vi "Configure Channel (Volt Log).vi"(0 "VISA resource name":refnum<visa-resource-name>, 1 "Scaling":T2={"Floating Point Position (2)"=2, "Lower Scaling (1.00E+0)"=1.0, "Upper Scaling (1.00E+2)"=100.0, "Unit Character (\"\")"=""} {"Upper Scaling (1.00E+2)" min=1e-15 max=1000000000000000.0 format="%.2e"; "Lower Scaling (1.00E+0)" min=1e-15 max=1000000000000000.0 format="%.2e"; "Floating Point Position (2)" min=1 max=2 step=1}, 5 "Channel (0001)":string="0001", 7 "Enable Channel (True)":bool=TRUE, 9 "Range And Span":T1={"Volt Range (4 : 2V)"=4, "Enable Span (False)"=FALSE, "Lower Span (2.0000)"=-2.0, "Upper Span (2.0000)"=2.0, "Bias (0)"=0.0} {"Upper Span (2.0000)" min=-99999.0 max=99999.0 step=1.0 format="%_5g"; "Lower Span (2.0000)" min=-99999.0 max=99999.0 step=1.0 format="%_5g"; "Volt Range (4 : 2V)" items=["20mV", "60mV", "200mV", "1V", "2V", "6V", "20V", "50V"]}, 11 "error in (no error)":errorcluster, 12 "Calculation (0: Log Input)":u16(ring) items=["Log Input", "Pseudo-log Input", "Linear-log Input"]) -> (4 "VISA resource name out":refnum<visa-resource-name>, 6 "Channel":string, 15 "error out":errorcluster)   [LabVIEW 2020, in "Yokogawa GX Series.lvlib"]
doc: "Sets the input range as voltage.\n\nCommand: SRangeAI"
uses:
  <instrlib>/Yokogawa GX Series/Yokogawa GX Series.lvlib
  <instrlib>/Yokogawa GX Series/Private/Volt Range.vi
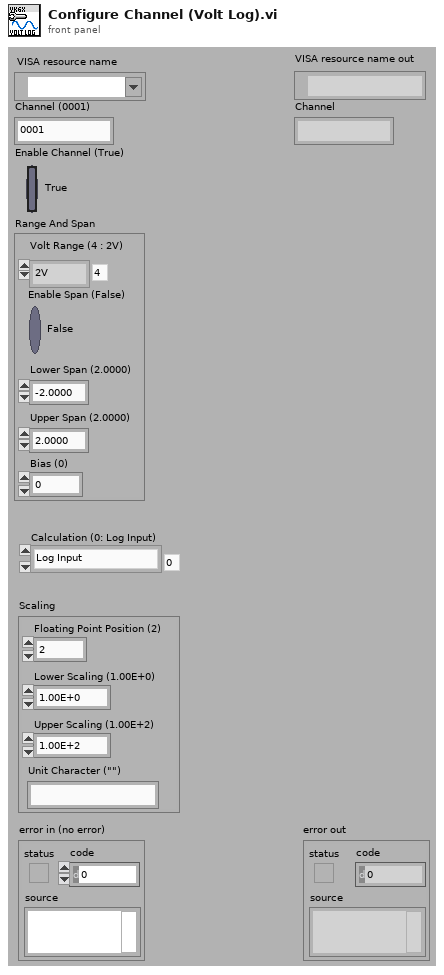
[diagram p1: front panel]
types:
  T1 = cluster{"Volt Range (4 : 2V)":i32, "Enable Span (False)":bool, "Lower Span (2.0000)":dbl, "Upper Span (2.0000)":dbl, "Bias (0)":dbl}
  T2 = cluster{"Floating Point Position (2)":i32, "Lower Scaling (1.00E+0)":dbl, "Upper Scaling (1.00E+2)":dbl, "Unit Character (\"\")":string}
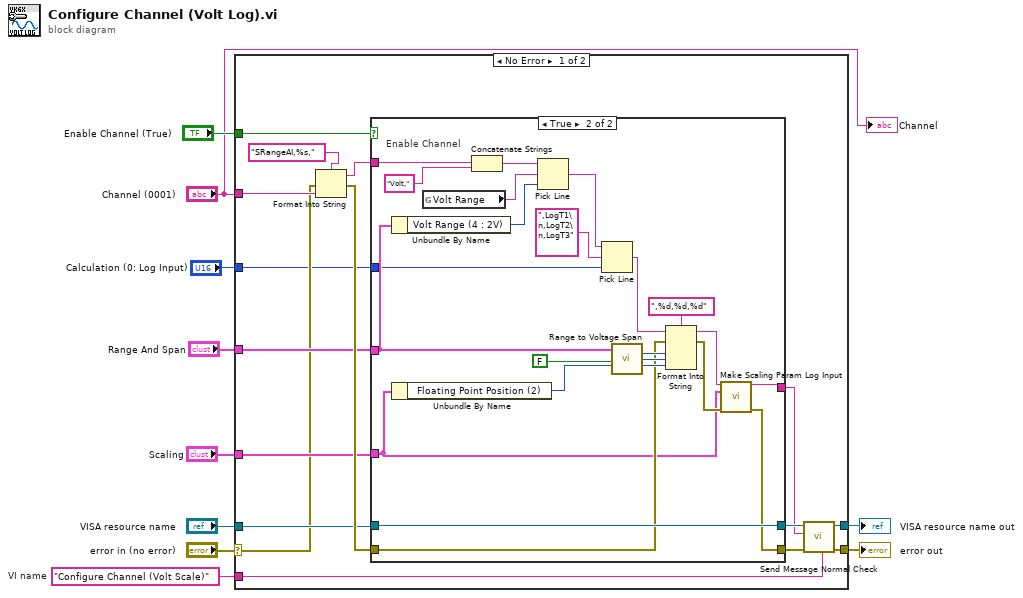
[diagram p0: block diagram]
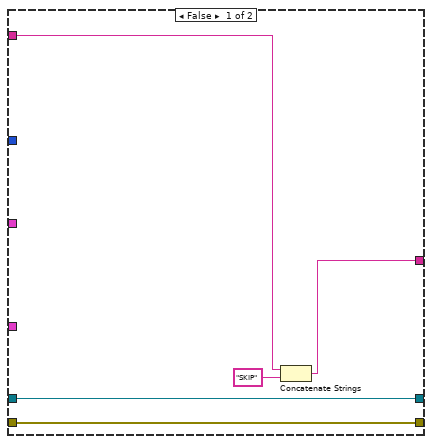
[diagram p2: hidden frame]
diagram:
  w6 = "Configure Channel (Volt Scale)"  # VI name
  n1 = case shown="No Error" "error in (no error)" {
    selector: "error in (no error)" -> [w12 w55]
    tunnel: "VISA resource name" -> [w23 w56]
    tunnel: "Scaling" -> [w22 _]
    tunnel: [w19 w56] -> w8
    tunnel: [w18 w55] -> w7
    tunnel: w6 -> [w16 _]
    tunnel: "Range And Span" -> [w15 _]
    tunnel: "Enable Channel (True)" -> [w14 _]
    tunnel: "Channel (0001)" -> [w13 _]
    tunnel: "Calculation (0: Log Input)" -> [w11 _]
    frame No Error {
      n2 = Format Into String(format string="SRangeAI,%s,", error in=w12, w13) -> (resulting string=w24:string, error out=w25:errorcluster)  [unwired: 1 in]
      n3 = case shown="True" w14 {
        tunnel: w25 -> [w28 w46]
        tunnel: [w28 w42] -> w20
        tunnel: w24 -> [w30 w53]
        tunnel: [w31 w40] -> w17
        tunnel: w23 -> [w27 w47]
        tunnel: [w27 w47] -> w21
        tunnel: w22 -> [_ w38]
        tunnel: w15 -> [_ w45]
        tunnel: w11 -> [_ w34]
        frame False {
          n4 = Concatenate Strings(w30, "SKIP") -> (w31:string)
        }
        frame True {
          # "Enable Channel"
          n5 = Unbundle By Name(w45) -> ("Volt Range (4 : 2V)"=w51:i32)
          n6 = Unbundle By Name(w38) -> ("Floating Point Position (2)"=w41:i32)
          n7 = global read "Volt Range.vi" "Volt Range"() -> (w36:string)
          n8 = Concatenate Strings(w53, "Volt,") -> (w52:string)
          n9 = Pick Line(string ("")=w52, multi-line string=w36, line index=w51) -> (output string=w35:string)
          n10 = Pick Line(string ("")=w35, multi-line string=",LogT1\n,LogT2\n,LogT3", line index=w34) -> (output string=w33:string)
          n11 = call <instrlib>:"Range to Voltage Span.vi"("Range And Span"=w45, "Scaling? (False)"=FALSE, "Floating Point Position (2)"=w41) -> ("Lower Span"=w50:i32, "Upper Span"=w49:i32, "Bias"=w48:i32)  [unwired: 5 in, 5 out]
          n12 = Format Into String(format string=",%d,%d,%d", initial string=w33, error in=w46, w50, w49, w48) -> (resulting string=w39:string, error out=w43:errorcluster)
          n13 = call <instrlib>:"Make Scaling Param Log Input.vi"("String (\"\")"=w39, "Scaling"=w38, "error in (no error)"=w43) -> ("String After"=w40:string, "error out"=w42:errorcluster)  [unwired: 11 in]
        }
      }
      n14 = call <instrlib>:"Send Message Normal Check.vi"("Source (\"\")"=w16, "error in (no error)"=w20, "Send Message (\"\")"=w17, "VISA resource name"=w21) -> ("error out"=w18:errorcluster, "VISA resource name out"=w19:refnum<visa-resource-name>)  [unwired: 2 in, 4 out]
    }
    frame Error {
    }
  }
  "error out" <- w7
  "VISA resource name out" <- w8
  "Channel" <- "Channel (0001)"
